vi "Remove_Source.vi"(8 "error in (no error)":errorcluster, 9 "source tag":string, 10 "source in":refnum<class "IB_Source.lvclass">[](array[class]), 11 "IB_DestTree in":refnum<class "IB_Tree_Dest.lvclass">) -> (0 "error out":errorcluster, 2 "source out":refnum<class "IB_Source.lvclass">[](array[class]), 3 "IB_DestTree out":refnum<class "IB_Tree_Dest.lvclass">)   [LabVIEW 2020, in "IB_Tree_Dest.lvclass"]
uses:
  <vilib>/AppBuilder/IB_Classes/Tree_Dest/IB_Tree_Dest.lvclass
  <vilib>/AppBuilder/IB_Classes/Tree_Dest/IB_Tree_Dest.lvclass/IB_Tree_Dest.ctl
  <vilib>/AppBuilder/IB_Classes/Tree/IB_Tree.lvclass
  <vilib>/AppBuilder/IB_Classes/Source/IB_Source.lvclass
  e:/builds/penguin/labview/branches/2020/dev/dist/vi.lib/AppBuilder/IB_Classes/Tree/IB_Tree.lvclass
  e:/builds/penguin/labview/branches/2020/dev/dist/vi.lib/AppBuilder/IB_Classes/Tree_Dest/IB_Tree_Dest.lvclass
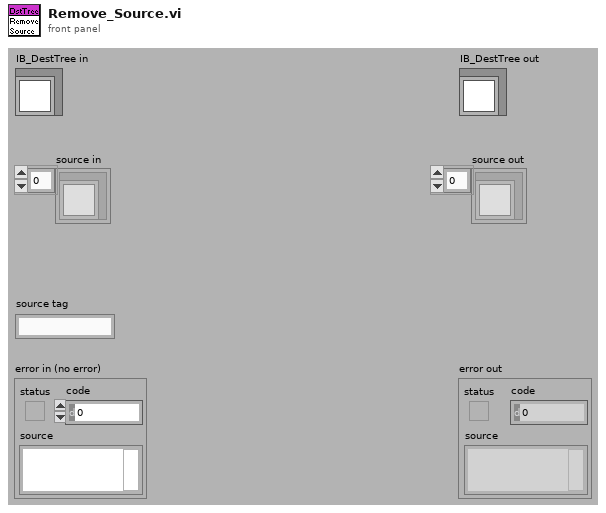
[diagram p1: front panel]
types:
  T1 = typedef "IB_Source.ctl" = cluster{"name":string, "sourceTag":string, "destTag":string, "path":path, "eng_installPath":string, "UI_inBuild?":bool, "str ref?":bool}
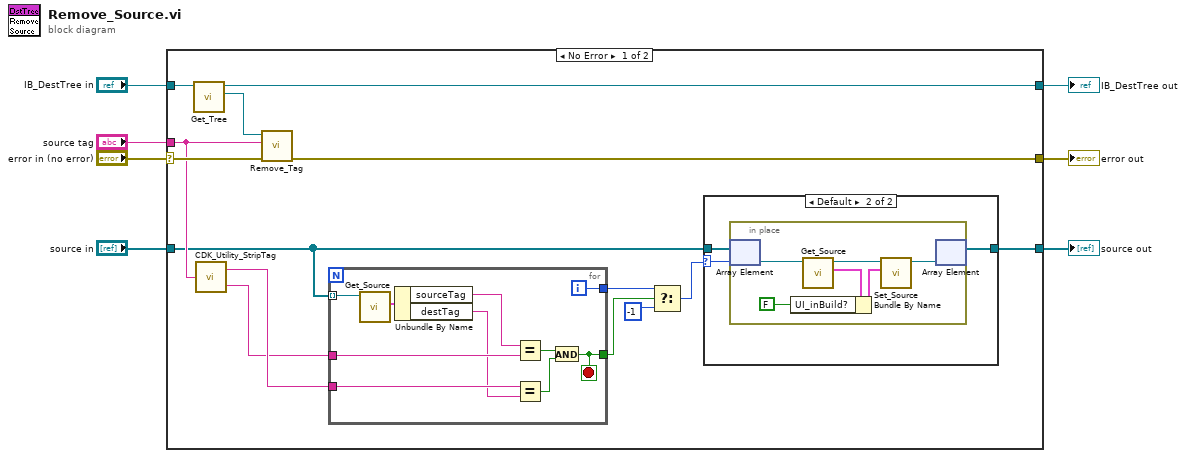
[diagram p0: block diagram]
diagram:
  n1 = case shown="No Error" "error in (no error)" {
    selector: "error in (no error)" -> [w18 w44]
    tunnel: [w17 w44] -> w6
    tunnel: [w20 w43] -> w4
    tunnel: "IB_DestTree in" -> [w21 w43]
    tunnel: "source tag" -> [w15 _]
    tunnel: "source in" -> [w11 w42]
    tunnel: [w16 w42] -> w1
    frame No Error {
      n2 = call <vilib>:"Get_Tree.vi"("IB_Tree in"=w21) -> ("ctl"=w19:refnum<vi>, "IB_Tree out"=w20:refnum<class "IB_Tree_Dest.lvclass">)  [unwired: 1 in, 8 out]
      n3 = call <resource>:"CDK_Utility_StripTag.vi"("Path"=w15) -> ("stripped path"=w10:string, "name"=w9:string)  [unwired: 1 in]
      n4 = call <vilib>:"Remove_Tag.vi"("error in"=w18, "tag"=w15, "Tree Refnum"=w19) -> ("error out"=w17:errorcluster)  [unwired: 3 in, 5 out]
      n5 = for {
        tunnel: w11 -> [w31] mode=indexing
        tunnel: w9 -> [w28]
        tunnel: w10 -> [w27]
        tunnel: [w23] -> w14
        tunnel: [w22] -> w13
        i -> [w22]
        stop <- w23 stop-if-true
        n6 = call <vilib>:"Get_Source.vi"("IB_Source in"=w31) -> ("data"=w30:T1)  [unwired: 1 in, 9 out]
        n7 = Unbundle By Name(w30) -> ("sourceTag"=w29:string, "destTag"=w26:string)
        n8 = Equal?(x=w29, y=w28) -> (x = y?=w25:bool)
        n9 = Equal?(x=w27, y=w26) -> (x = y?=w24:bool)
        n10 = And(x=w25, y=w24) -> (x .and. y?=w23:bool)
      }
      n11 = Select(t=w13, s=w14, f=-1) -> (s? t:f=w8:i32)
      n12 = case shown="Default" w8 {
        selector: w8 -> [_ w33]
        tunnel: w11 -> [w32 w35]
        tunnel: [w32 w34] -> w16
        frame -1 {
        }
        frame Default {
          n13 = in-place {
            n14 = in-place-array #1(w35, w33) -> (w41:refnum<class "IB_Source.lvclass">)
            n15 = call <vilib>:"Get_Source.vi"("IB_Source in"=w41) -> ("data"=w38:T1, "IB_Source out"=w39:refnum<class "IB_Source.lvclass">)  [unwired: 1 in, 8 out]
            n16 = Bundle By Name(cluster=w38, "UI_inBuild?"=FALSE) -> (w37:T1)
            n17 = call <vilib>:"Set_Source.vi"("data"=w37, "IB_Source in"=w39) -> ("IB_Source out"=w40:refnum<class "IB_Source.lvclass">)  [unwired: 1 in, 8 out]
            n18 = in-place-array #1(w40) -> (w34:refnum<class "IB_Source.lvclass">[])  [unwired: 1 out]
          }
        }
      }
    }
    frame Error {
    }
  }
  "error out" <- w6
  "IB_DestTree out" <- w4
  "source out" <- w1
